vi "OPC UA Read.vi"() -> ()   [LabVIEW 2023]
uses:
  <vilib>/OPCUA/client/Multiple Read Double.vi
  <vilib>/OPCUA/NI OPC UA Client.lvlib
panel:
  out "Temperature Value":dbl format="%#.2g"
  in  "Node ID":string
  in  "stop":bool
  in  "server endpoint URL":string
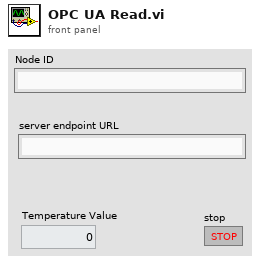
[diagram p1: front panel]
types:
  T1 = cluster{"message mode":enum16{"None", "Sign", "Sign and Encrypt"}, "security":enum16{"Basic256", "Basic128Rsa15"}}
  T2 = typedef "OPC UA Client Refnum.ctl" = refnum<k21>
  T3 = typedef "NodeId.ctl" = string
  T4 = typedef "OPC UA StatusCode.ctl" = u32
  T5 = cluster{"node ID":T3, "value ":dbl, "timestamp":timestamp, "status":T4}[]
  T6 = cluster{"node ID":T3, "value ":dbl, "timestamp":timestamp, "status":T4}
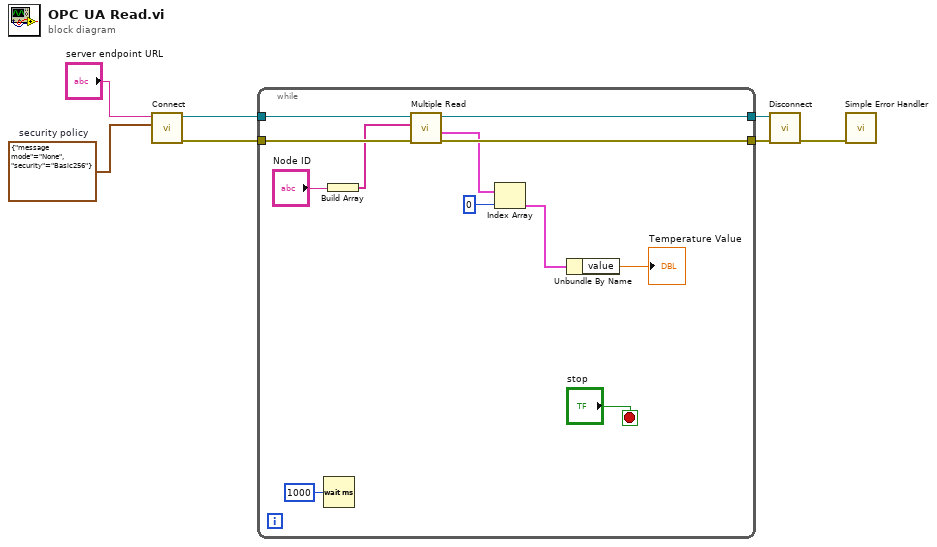
[diagram p0: block diagram]
diagram:
  w1 = T1 {"message mode"=enum."None", "security"=enum."Basic256"}  # security policy
  n1 = call <vilib>:"Connect.vi"("security policy"=w1, "server endpoint URL"="server endpoint URL") -> ("error out"=w6:errorcluster, "OPC UA client refnum out"=w4:T2)  [unwired: 7 in, 1 out]
  n2 = while {
    tunnel: w6 -> [w17]
    tunnel: [w16] -> w5
    tunnel: w4 -> [w15]
    tunnel: [w14] -> w3
    stop <- "stop" stop-if-true
    n3 = Wait (ms)(milliseconds to wait=u32 1000) -> ()  [unwired: 1 out]
    n4 = Build Array("Node ID") -> (w12:string[])
    n5 = call-poly <vilib>:"Multiple Read.vi"("error in (no error)"=w17, "node IDs"=w12, "OPC UA client refnum in"=w15) -> ("error out"=w16:errorcluster, "results"=w11:T5, "OPC UA client refnum out"=w14:T2)  [unwired: 5 in, 1 out]
    n6 = Index Array(array=w11, index=0) -> (element=w9:T6)
    n7 = Unbundle By Name(w9) -> ("value"=→"Temperature Value":dbl)
  }
  n8 = call <vilib>:"Disconnect.vi"("error in (no error)"=w5, "OPC UA client refnum in"=w3) -> ("error out"=w7:errorcluster)  [unwired: 9 in]
  n9 = call <vilib>:"Simple Error Handler.vi"("error in (no error)"=w7) -> ()  [unwired: 4 in, 5 out]
